vi "FindInstruments.vi"(8 "error in (no error)":errorcluster, 10 "InstrumentData":T1, 11 "ZWO_ASI in":refnum<class "ZWO_ASI.lvclass">) -> (0 "error out":errorcluster, 3 "ZWO_ASI out":refnum<class "ZWO_ASI.lvclass">)   [LabVIEW 2023, in "ZWO_ASI.lvlib" / "ZWO_ASI.lvclass"]
uses:
  ZWO_ASI.lvclass
  Labview_ASI_demo_64bit_221128/user.lib/ASICamera2_no_err/ASICamera2_no_err.lvlib
  typedefs/instrumentType.ctl
  typedefs/typedefs.lvlib
  <vilib>/ActorFramework/Actor/Actor.lvclass
  C:/Program Files/National Instruments/LabVIEW 2023/vi.lib/ActorFramework/Actor/Actor.lvclass
  C:/Users/quantum/Documents/LVDAQ/ConcreteClasses/ConcreteInstrumentClasses/CameraClasses/ZWO_ASI_LV/ZWO_ASI/ZWO_ASI.lvclass
  C:/Users/quantum/Documents/LVDAQ/Interfaces/AbstractInstrumentClasses/Cameras_LV/CameraInterface/CameraInterface.lvclass
  C:/Users/quantum/Documents/LVDAQ/Interfaces/InitDeinitInterface/InitDeinit/InitDeinit.lvclass
  <vilib>/ActorFramework/Message Enqueuer/Message Enqueuer.lvclass
  typedefs/InstrumentData.ctl
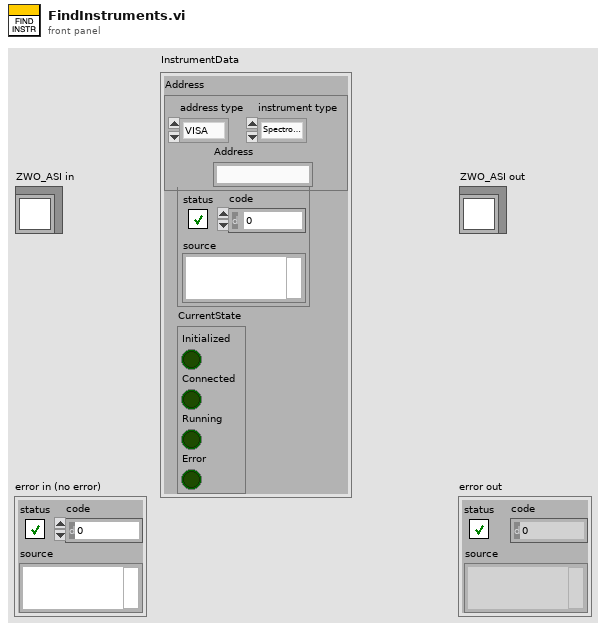
[diagram p1: front panel]
types:
  T1 = typedef "typedefs.lvlib/InstrumentData.ctl" = cluster{"Instr Error":errorcluster, "Address":cluster{"address type":enum16{"VISA", "Index"}, "Address":string, "instrument type":T2}, "CurrentState":cluster{"Initialized":bool, "Connected":bool, "Running":bool, "Error":bool}}
  T2 = typedef "typedefs.lvlib/instrumentType.ctl" = enum16{"Spectrometer", "Camera", "Stepper", "Piezo", "SLM"}
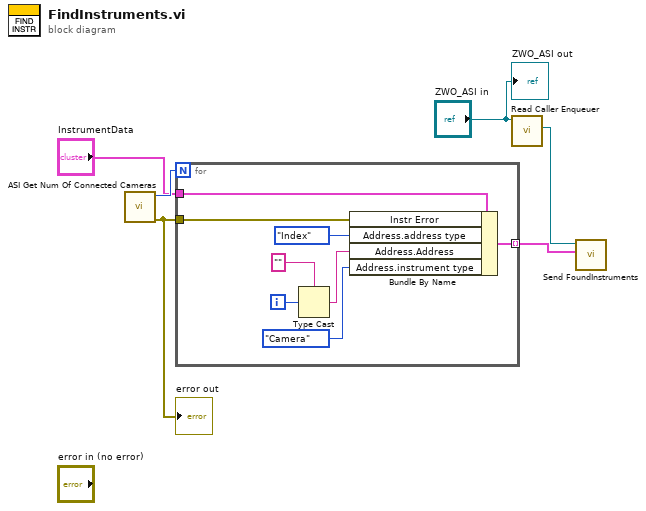
[diagram p0: block diagram]
diagram:
  n1 = call "ASI Get Num Of Connected Cameras.vi"() -> ("error out"=w6:errorcluster, "function return"=w5:i32)  [unwired: 10 in]
  "error out" <- w6
  n2 = for {
    N: w5 -> [_]
    tunnel: w6 -> [w14]
    tunnel: [w8] -> w1 mode=indexing
    tunnel: "InstrumentData" -> [w7]
    i -> [w10]
    n3 = Type Cast(type="", x=w10) -> (*(type *) &x=w9:string)
    n4 = Bundle By Name(cluster=w7, "Instr Error"=w14, "Address.address type"=enum16{"VISA", "Index"}."Index", "Address.Address"=w9, "Address.instrument type"=instrumentType."Camera") -> (w8:T1)
  }
  n5 = call <vilib>:"Read Caller Enqueuer.vi"("Actor"="ZWO_ASI in") -> ("Caller Enqueuer"=w4:refnum<class "Message Enqueuer.lvclass">)  [unwired: 10 in]
  n6 = call "Send FoundInstruments.vi"("FoundInstruments"=w1, "Message Enqueuer"=w4) -> ()  [unwired: 8 in, 2 out]
  "ZWO_ASI out" <- "ZWO_ASI in"
